vi "Task Type.vi"(11 "RemoteMessaging in":refnum<class "RemoteMessaging.lvclass">) -> (2 "Task Type":string)   [LabVIEW 2020, in "Volatus.lvlib" / "RemoteMessaging.lvclass"]
uses:
  RemoteMessaging.lvclass
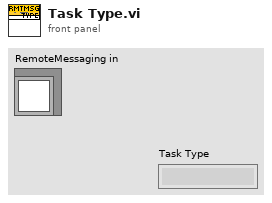
[diagram p1: front panel]
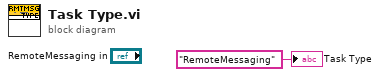
[diagram p0: block diagram]
diagram:
  "Task Type" <- "RemoteMessaging" ("Task Type")
